vi "读取内置参数.vi"(8 "error in (no error)":errorcluster, 11 "MB session in":refnum<class "MB_Master.lvclass">) -> (0 "error out":errorcluster, 1 "float":T1 {"偏心轮校准参数" format="%#.6g"}, 2 "外设配置":T3 {"是否存在液位检测板" items=["否", "是"]; "阀数量" items=["9通"=9, "12通"=12]; "泵类型" items=["TECAN", "润泽"]}, 3 "MB session out":refnum<class "MB_Master.lvclass">, 5 "量程参数读取":T2 {"阈值（高->低）" format="%#.6g"; "阈值（低->高）" format="%#.6g"; "下限" format="%#.6g"; "上限" format="%#.6g"})   [LabVIEW 2016, in "斯坦道CODMn新电路板.lvlib"]
uses:
  <vilib>/Plasmionique/MB Master/MB_Master/MB_Master.lvclass
  <vilib>/Plasmionique/MB Master/MB_Master_Serial/MB_Master_Serial.lvclass
  C:/Program Files (x86)/National Instruments/LabVIEW 2016/vi.lib/Plasmionique/MB Master/MB_Master/MB_Master.lvclass
  <vilib>/Plasmionique/MB Master/MB Master.lvlib
panel:
  in  "VISA Resource":refnum<visa-resource-name>
  in  "引用选择":enum16{"MB引用", "自建引用"}(ring)
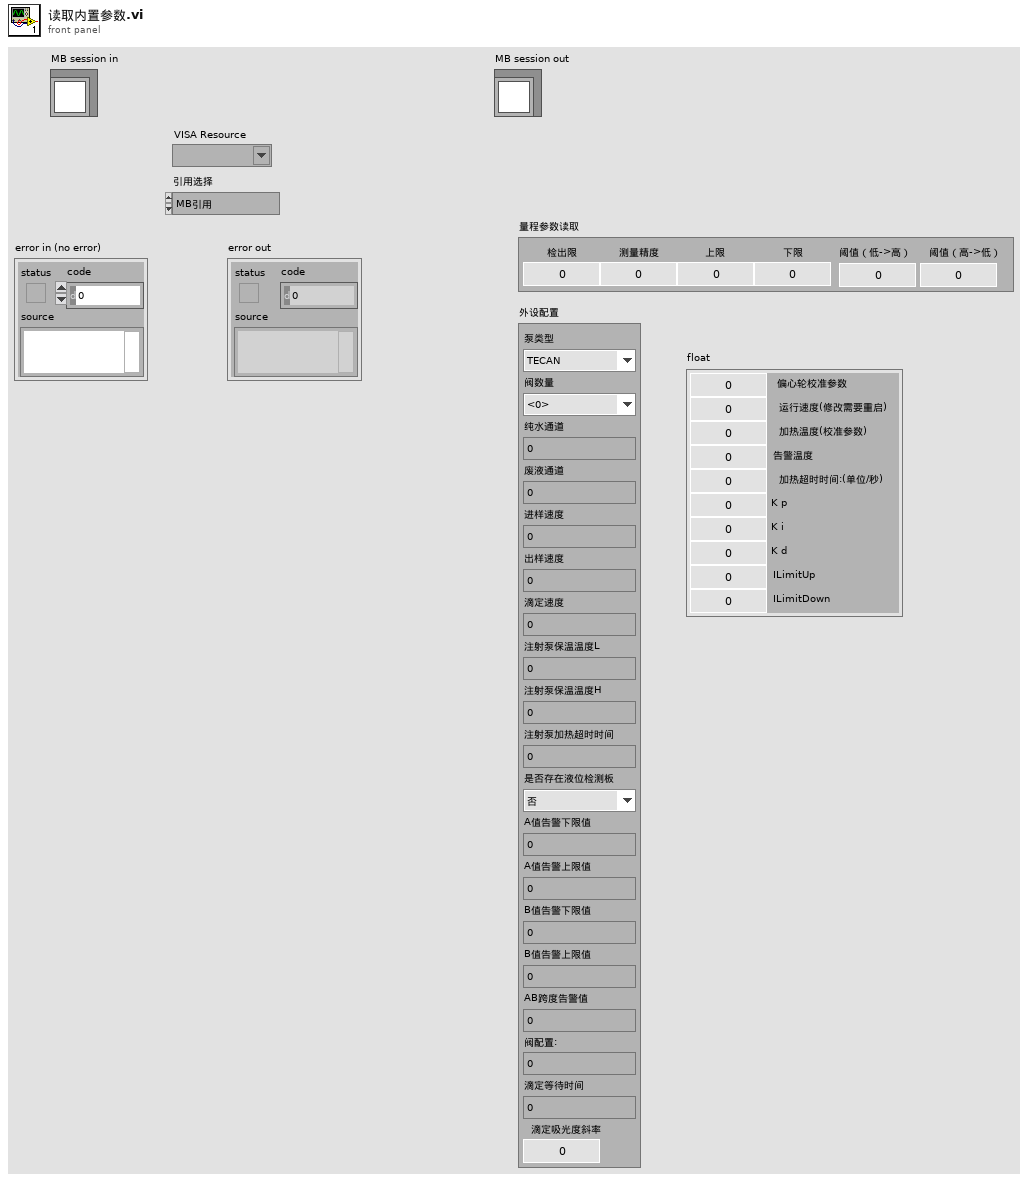
[diagram p1: front panel]
types:
  T1 = cluster{"偏心轮校准参数":dbl, "运行速度(修改需要重启)":u16, "加热温度(校准参数) ":dbl, "告警温度":dbl, "加热超时时间:(单位/秒)":dbl, "K p":dbl, "K i":dbl, "K d":dbl, "ILimitUp":dbl, "ILimitDown":dbl}
  T2 = cluster{"检出限":dbl, "测量精度":dbl, "上限":dbl, "下限":dbl, "阈值（低->高）":dbl, "阈值（高->低）":dbl}
  T3 = cluster{"泵类型":u8, "阀数量":u8, "纯水通道":u8, "废液通道":u8, "进样速度":u16, "出样速度":u16, "滴定速度":u16, "注射泵保温温度L":u8, "注射泵保温温度H":u8, "注射泵加热超时时间":u16, "是否存在液位检测板":u16, "A值告警下限值":u16, "A值告警上限值":u16, "B值告警下限值":u16, "B值告警上限值":u16, "AB跨度告警值":u16, "阀配置:":u8, "滴定等待时间":u16, "滴定吸光度斜率":dbl}
  T4 = cluster{"baud rate (bps)":u32, "stop bits":u16, "parity":u16, "flow control":u16, "timeout":u32, "retries":i32}
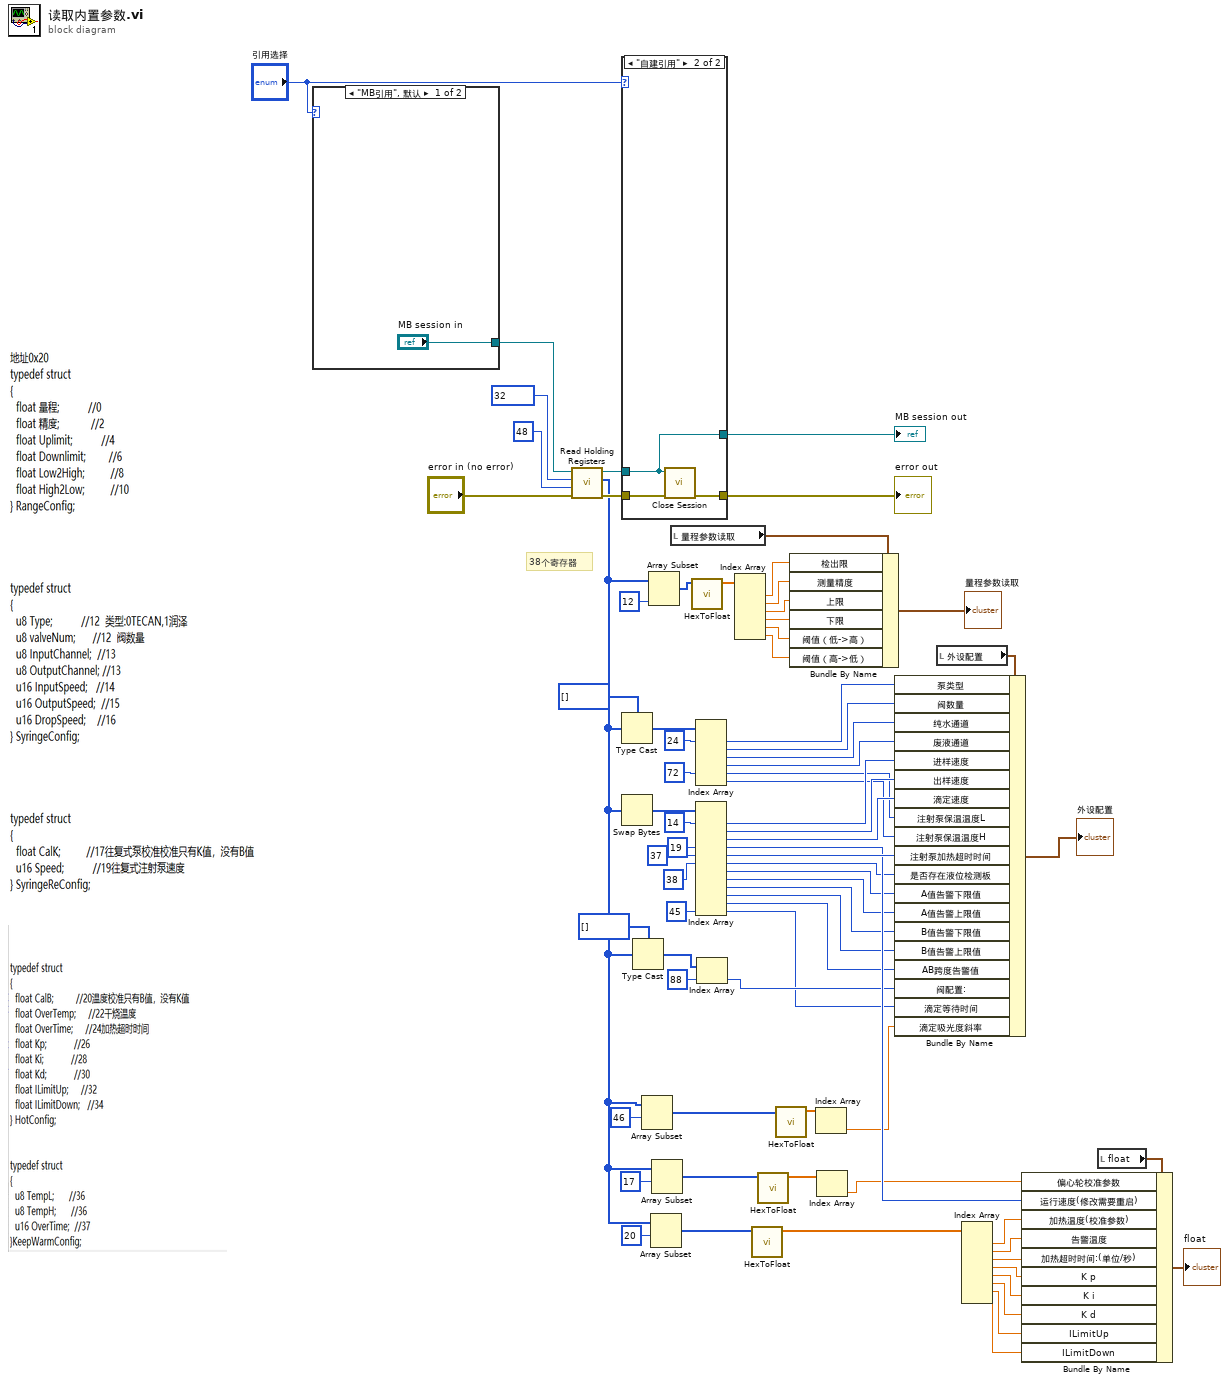
[diagram p0: block diagram]
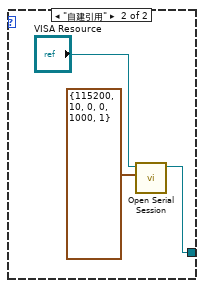
[diagram p3: hidden frame]
diagram:
  # "38个寄存器"
  n1 = case shown="\"MB引用\", 默认" "引用选择" {
    tunnel: ["MB session in" w80] -> w68
    frame "MB引用", Default {
    }
    frame "自建引用" {
      n2 = call <vilib>:"Open Serial Session.vi"("Serial Config"=T4 {"baud rate (bps)"=115200, "stop bits"=10, "parity"=0, "flow control"=0, "timeout"=1000, "retries"=1}, "VISA Resource"="VISA Resource") -> ("MB_Serial session"=w80:refnum<class "MB_Master_Serial.lvclass">)  [unwired: 8 in, 1 out]
    }
  }
  n3 = call <vilib>:"Read Holding Registers.vi"("error in (no error)"="error in (no error)", "quantity"=u16 48, "starting address"=u16 32, "MB session in"=w68) -> ("error out"=w65:errorcluster, "Registers"=w2:u16[], "MB session out"=w67:refnum<class "MB_Master.lvclass">)  [unwired: 5 in]
  n4 = case shown="\"自建引用\"" "引用选择" {
    tunnel: w67 -> [w81 w83]
    tunnel: w65 -> [w82 w85]
    tunnel: [w82 w84] -> w64
    tunnel: [w81 w83] -> w63
    frame "MB引用", Default {
    }
    frame "自建引用" {
      n5 = call-dynamic "Close Session.vi"("error in (no error)"=w85, "MB session in"=w83) -> ("error out"=w84:errorcluster)  [unwired: 9 in]
    }
  }
  "MB session out" <- w63
  "error out" <- w64
  n6 = Type Cast(type=u8[] [], x=w2) -> (*(type *) &x=w69:u8[])
  n7 = Swap Bytes(anything=w2) -> (byte swapped=w42:u16[])
  n8 = Type Cast(type=u8[] [], x=w2) -> (*(type *) &x=w5:u8[])
  n9 = Array Subset(array=w2, index=46 ("索引")) -> (w1:u16[])  [unwired: 1 in]
  n10 = Array Subset(array=w2, length=12 ("长度")) -> (w24:u16[])  [unwired: 1 in]
  n11 = Array Subset(array=w2, index=20 ("索引")) -> (w22:u16[])  [unwired: 1 in]
  n12 = Array Subset(array=w2, index=17 ("索引")) -> (w35:u16[])  [unwired: 1 in]
  n13 = local read "量程参数读取"() -> (w61:T2)
  n14 = call "HexToFloat.vi"("数组"=w24) -> ("FLOAT"=w62:sgl[])  [unwired: 10 in]
  n15 = Index Array(array=w69, index #1=24 ("索引"), index #5=72 ("索引")) -> (element #1=w70:u8, element #2=w53:u8, element #3=w52:u8, element #4=w51:u8, element #5=w46:u8, element #6=w45:u8)  [unwired: 4 in]
  n16 = Index Array(array=w42, index #1=14 ("索引"), index #4=19 ("索引"), index #5=37 ("索引"), index #6=38 ("索引"), index #12=45 ("索引")) -> (element #1=w50:u16, element #2=w49:u16, element #3=w48:u16, element #4=w34:u16, element #5=w39:u16, element #6=w18:u16, element #7=w16:u16, element #8=w15:u16, element #9=w14:u16, element #10=w13:u16, element #11=w12:u16, element #12=w3:u16)  [unwired: 7 in]
  n17 = Index Array(array=w5, index=88 ("索引")) -> (element=w9:u8)
  n18 = Index Array(array=w62) -> (element #1=w59:sgl, element #2=w58:sgl, element #3=w57:sgl, element #4=w56:sgl, element #5=w55:sgl, element #6=w54:sgl)  [unwired: 6 in]
  n19 = call "HexToFloat.vi"("数组"=w22) -> ("FLOAT"=w21:sgl[])  [unwired: 10 in]
  n20 = call "HexToFloat.vi"("数组"=w35) -> ("FLOAT"=w20:sgl[])  [unwired: 10 in]
  n21 = call "HexToFloat.vi"("数组"=w1) -> ("FLOAT"=w8:sgl[])  [unwired: 10 in]
  n22 = Bundle By Name(cluster=w61, "检出限"=w59, "测量精度"=w58, "上限"=w57, "下限"=w56, "阈值（低->高）"=w55, "阈值（高->低）"=w54) -> (→"量程参数读取":T2)
  n23 = Index Array(array=w8) -> (element=w6:sgl)  [unwired: 1 in]
  n24 = Index Array(array=w20) -> (element=w19:sgl)  [unwired: 1 in]
  n25 = local read "外设配置"() -> (w72:T3)
  n26 = Bundle By Name(cluster=w72, "泵类型"=w70, "阀数量"=w53, "纯水通道"=w52, "废液通道"=w51, "进样速度"=w50, "出样速度"=w49, "滴定速度"=w48, "注射泵保温温度L"=w46, "注射泵保温温度H"=w45, "注射泵加热超时时间"=w39, "是否存在液位检测板"=w18, "A值告警下限值"=w16, "A值告警上限值"=w15, "B值告警下限值"=w14, "B值告警上限值"=w13, "AB跨度告警值"=w12, "阀配置:"=w9, "滴定等待时间"=w3, "滴定吸光度斜率"=w6) -> (→"外设配置":T3)
  n27 = Index Array(array=w21) -> (element #1=w33:sgl, element #2=w32:sgl, element #3=w31:sgl, element #4=w30:sgl, element #5=w29:sgl, element #6=w28:sgl, element #7=w27:sgl, element #8=w26:sgl)  [unwired: 8 in]
  n28 = local read "float"() -> (w38:T1)
  n29 = Bundle By Name(cluster=w38, "偏心轮校准参数"=w19, "运行速度(修改需要重启)"=w34, "加热温度(校准参数)"=w33, "告警温度"=w32, "加热超时时间:(单位/秒)"=w31, "K p"=w30, "K i"=w29, "K d"=w28, "ILimitUp"=w27, "ILimitDown"=w26) -> (→"float":T1)
